vi "parseStatus.vi"(8 "error in (no error)":errorcluster, 10 "response":string, 11 "IResponseParser in":refnum<class "IResponseParser.lvclass">) -> (0 "error out":errorcluster, 2 "status":string, 3 "IResponseParser out":refnum<class "IResponseParser.lvclass">)   [LabVIEW 2023, in "AbstractFactory.lvlib" / "IResponseParser.lvclass"]
uses:
  IResponseParser.lvclass
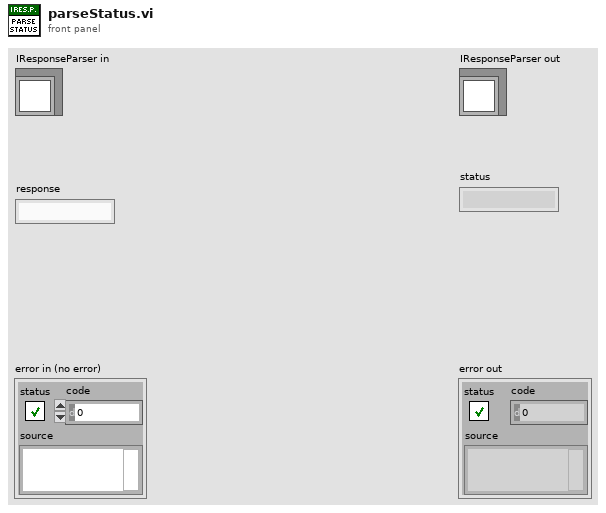
[diagram p1: front panel]
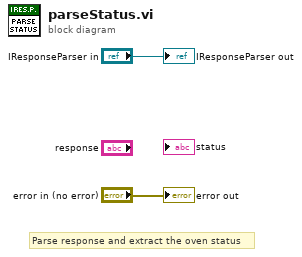
[diagram p0: block diagram]
diagram:
  # "Parse response and extract the oven status"
  "error out" <- "error in (no error)"
  "IResponseParser out" <- "IResponseParser in"
